vi "4_Analog_Meter_Reader(Inference)_(Input_From_File).vi"() -> ()   [LabVIEW 2020]
uses:
  Controls/Analog_Meter.ctl
  <vilib>/Ngene/Deep Learning Toolkit/Toolkit/NN_Network/Controls/NN_Save_Before_Destroy_Options.ctl
  <vilib>/Ngene/Deep Learning Toolkit/Toolkit/NN_Network/Controls/NN_Device.ctl
  <vilib>/Ngene/Deep Learning Toolkit/Toolkit/NN_Network/API/NN_Set_Input/3D/NN_Set_Input(3D_SGL_idx).vi
  <vilib>/Ngene/Deep Learning Toolkit/Toolkit/Deep_Learning_Toolkit_by_Ngene.lvlib
  <vilib>/ptbypt/NI_PtbyPt.lvlib
  <vilib>/vision/NI_Vision_Development_Module.lvlib
panel:
  out "Image Path":path=path "D:/working/Analog_Meter/Test/Images/0016.png"
  in  "File Path":path=path "D:/working/Analog_Meter/Test/Images/0016.png"
  out "Input":T1(plugin-control)
  out "Value":sgl=11.692846 format="%#.2g"
  out "Inference Time (ms)":dbl=0.008072819999924832 format="%#_3p"
  out "Prediction":T2=11.692846298217773 scale=0.0..140.0
  out "Inference Speed (FPS)":dbl=123.87245101579265 format="%#_3p"
  in  "Stop":bool
  in  "Network Configuration File Path":path=path "D:/Ngene/GitHub/deepltk_examples/3_Image_Processing/31_Image_Regression/working/Analog_Meter/Analog_Meter_net_cfg_24_01_29__19_35_37.cfg"
  in  "Weight File Path":path=path "D:/Ngene/GitHub/deepltk_examples/3_Image_Processing/31_Image_Regression/working/Analog_Meter/Analog_Meter_weights_24_01_29__19_35_37.bin"
  # "Instructions:\n1. Provide model files (.cfg and .bin).\n2. Run the VI\n3. Specify (Drag and Drop) an image from Test dataset in \"Input\" file path."
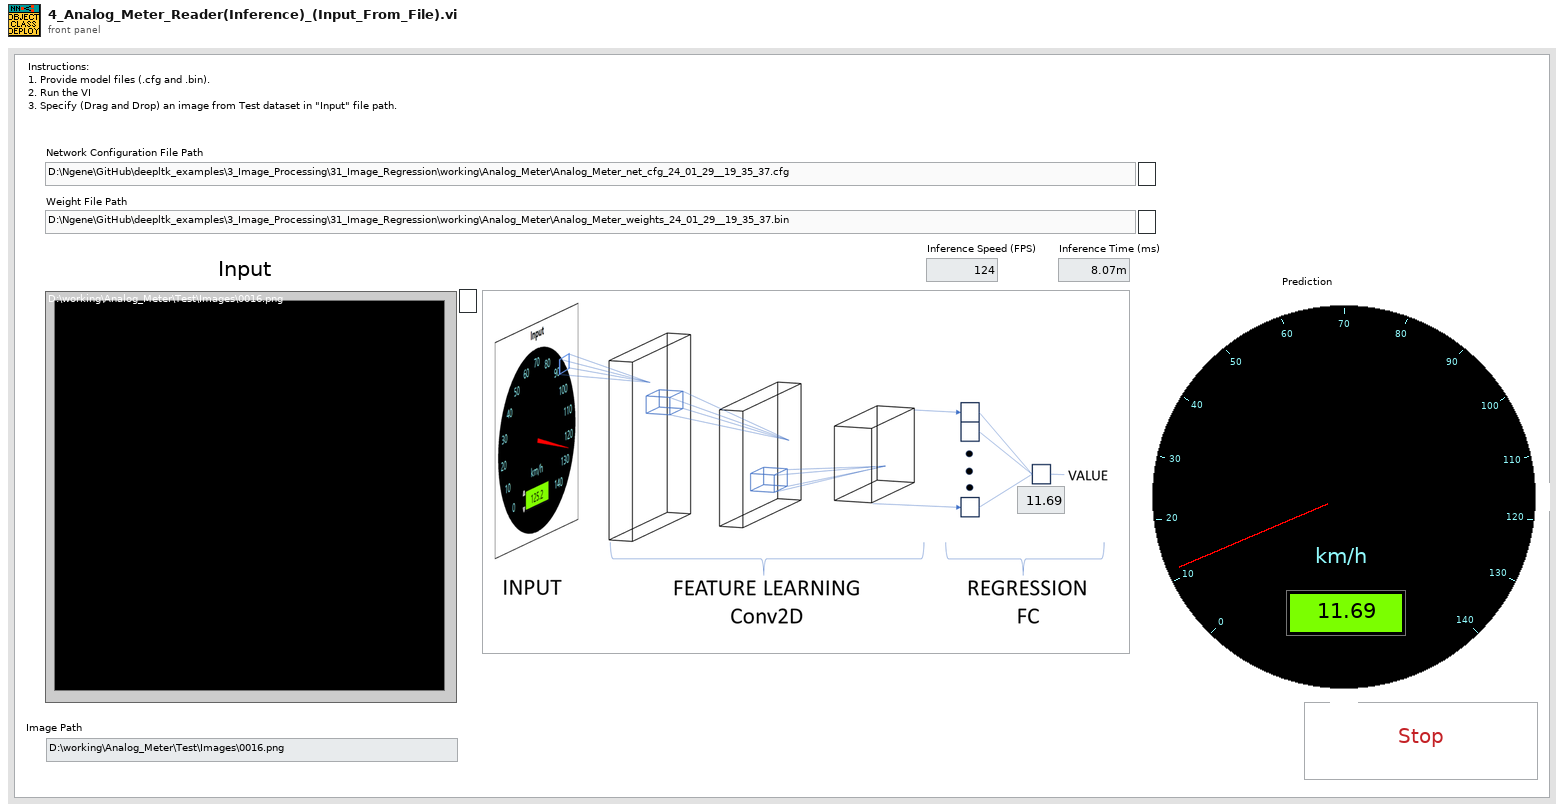
[diagram p1: front panel]
types:
  T1 = typedef "IMAQ Image.ctl" = refnum<image>
  T2 = typedef "Analog_Meter.ctl" = dbl
  T3 = typedef "Image Type" = u32
  T4 = typedef "Deep_Learning_Toolkit_by_Ngene.lvlib/NN_Device.ctl" = enum16{"CPU", "GPU"}
  T5 = typedef "Deep_Learning_Toolkit_by_Ngene.lvlib/NN_Save_Before_Destroy_Options.ctl" = cluster{"CFG?":bool, "Weights?":bool, "Render?":bool}
  T6 = typedef "Deep_Learning_Toolkit_by_Ngene.lvlib/NN_Config_Params.ctl" = cluster{"Name":string, "mBatch":i32, "NN_Train_Params":T7, "LR_Decay_Policy":T10, "Labels":string[], "Loss":T12}
  T7 = typedef "Deep_Learning_Toolkit_by_Ngene.lvlib/NN_Train_Params.ctl" = cluster{"Optimizer":T8, "Beta_1":sgl, "Beta_2":sgl, "Weight Decay(L1)":sgl, "Weight Decay(L2)":sgl, "Data_Sampling":T9}
  T8 = typedef "Deep_Learning_Toolkit_by_Ngene.lvlib/NN_Train_Optimizer.ctl" = enum16{"SGD", "Adam", "Adagrad", "Adadelta", "RMSProp", "Nesterov"}
  T9 = typedef "Deep_Learning_Toolkit_by_Ngene.lvlib/NN_Train_Data_Sampling.ctl" = enum16{"Random", "Sequential"}
  T10 = typedef "Deep_Learning_Toolkit_by_Ngene.lvlib/NN_LR_Policy_Cfg.ctl" = cluster{"Policy_Type":T11, "LR0":dbl, "k":sgl, "WarmUp_Policy":enum16{"Step", "Ramp"}, "WarmUp_Iter":i32, "WarmUp_Ratio":sgl}
  T11 = typedef "Deep_Learning_Toolkit_by_Ngene.lvlib/NN_LR_Policy_Type.ctl" = enum16{"Manual", "Step", "Exp", "1/t"}
  T12 = typedef "Deep_Learning_Toolkit_by_Ngene.lvlib/NN_Loss_Config_Params.ctl" = cluster{"Loss_Type":T13, "Loss_Conf_Params":variant}
  T13 = typedef "Deep_Learning_Toolkit_by_Ngene.lvlib/NN_Loss_Type.ctl" = enum16{"None", "MSE", "CrossEntropy", "YOLO_v2", "YOLO_v4"}
  T14 = typedef "Deep_Learning_Toolkit_by_Ngene.lvlib/NN_Layer_Config_Params.ctl" = cluster{"Layer_Type":T15, "Layer_Conf_Params":variant, "Input Layers":string[]}
  T15 = typedef "Deep_Learning_Toolkit_by_Ngene.lvlib/NN_Layer_Type.ctl" = enum16{"Input1D", "Input3D", "Conv1D", "Conv2D", "Conv2D_Adv", "MaxPool", "AvgPool", "UpSample", "DropOut3D", "ShortCut", "Concat", "SoftMax3D", "FC", "DropOut", "Softmax", "Flatten", "YOLO_v2", "YOLO_v4", "Activation", "BatchNormalization", "Unsupported"}
  T16 = typedef "Deep_Learning_Toolkit_by_Ngene.lvlib/NN.ctl" = cluster{"Name":string, "No of Layers":i32, "mBatch":i32, "Layers":T17[], "Dimty":T18, "Dims_In":T19, "Dims_Out":T19, "Working_Dir":path, "Train?":bool, "Train_Params":T7, "LR_Update_Policy":T10, "Session Data":T20, "Ground_truth":T21, "NNg_hdls":T22, "NN_Device":T4, "GPU Id":i32, "Labels":string[], "Receptive Field":T23[], "Loss_Type":T13, "Loss_Cfg_Prms":variant, "NNG_WS":T24}
  T17 = typedef "Deep_Learning_Toolkit_by_Ngene.lvlib/NN_Layer_ref.ctl" = refnum<data-value>
  T18 = typedef "Deep_Learning_Toolkit_by_Ngene.lvlib/NN_In_Out_Dim-ty.ctl" = enum8{"In1D_Out1D", "In3D_Out1D", "In3D_Out3D", "In3D_OutBBox"}
  T19 = typedef "Deep_Learning_Toolkit_by_Ngene.lvlib/NN_Dims(C,H,W).ctl" = cluster{"C":i32, "H":i32, "W":i32}
  T20 = typedef "Deep_Learning_Toolkit_by_Ngene.lvlib/NN_Train_Session_Data.ctl" = cluster{"Epochs":sgl, "Tot_Iter":i32, "LR":sgl, "LR_iter":i32}
  T21 = typedef "Deep_Learning_Toolkit_by_Ngene.lvlib/NN_Ground_truth.ctl" = cluster{"Y":variant}
  T22 = typedef "Deep_Learning_Toolkit_by_Ngene.lvlib/nng_cuda_handles.ctl" = cluster{"cudnn":u64, "cublas":u64, "stream":u64, "curand":u64}
  T23 = typedef "Deep_Learning_Toolkit_by_Ngene.lvlib/NN_Dims(V,H).ctl" = cluster{"V":i32, "H":i32}
  T24 = typedef "Deep_Learning_Toolkit_by_Ngene.lvlib/NNG_WS.ctl" = cluster{"NNG_WS_Mem":T25, "Max_WS_Size":i64}
  T25 = typedef "Deep_Learning_Toolkit_by_Ngene.lvlib/NNg_WS_Mem_DVR.ctl" = refnum<data-value>
  T26 = typedef "Deep_Learning_Toolkit_by_Ngene.lvlib/NN_Layer.ctl" = cluster{"Name":string, "Layer_Data":variant, "Layer_Type":T15, "Dims_In":T19, "Layers_In":variant, "Dims_Out":T19, "Layers_Out":variant, "Metrics":T27, "GPU_Data":variant, "mBatch":i32, "NN_Device":T4, "NNg_hdls":T22, "Train?":bool, "Dimty":T28, "RecptField":T29}
  T27 = typedef "Deep_Learning_Toolkit_by_Ngene.lvlib/NN_Layer_Metrics.ctl" = cluster{"Data":dbl, "Params":dbl, "Ops":dbl}
  T28 = typedef "Deep_Learning_Toolkit_by_Ngene.lvlib/NN_Layer_Dimty.ctl" = enum16{"1D", "3D"}
  T29 = typedef "Deep_Learning_Toolkit_by_Ngene.lvlib/NN_Layer_RF_State.ctl" = cluster{"Dims":T23, "J":T23}
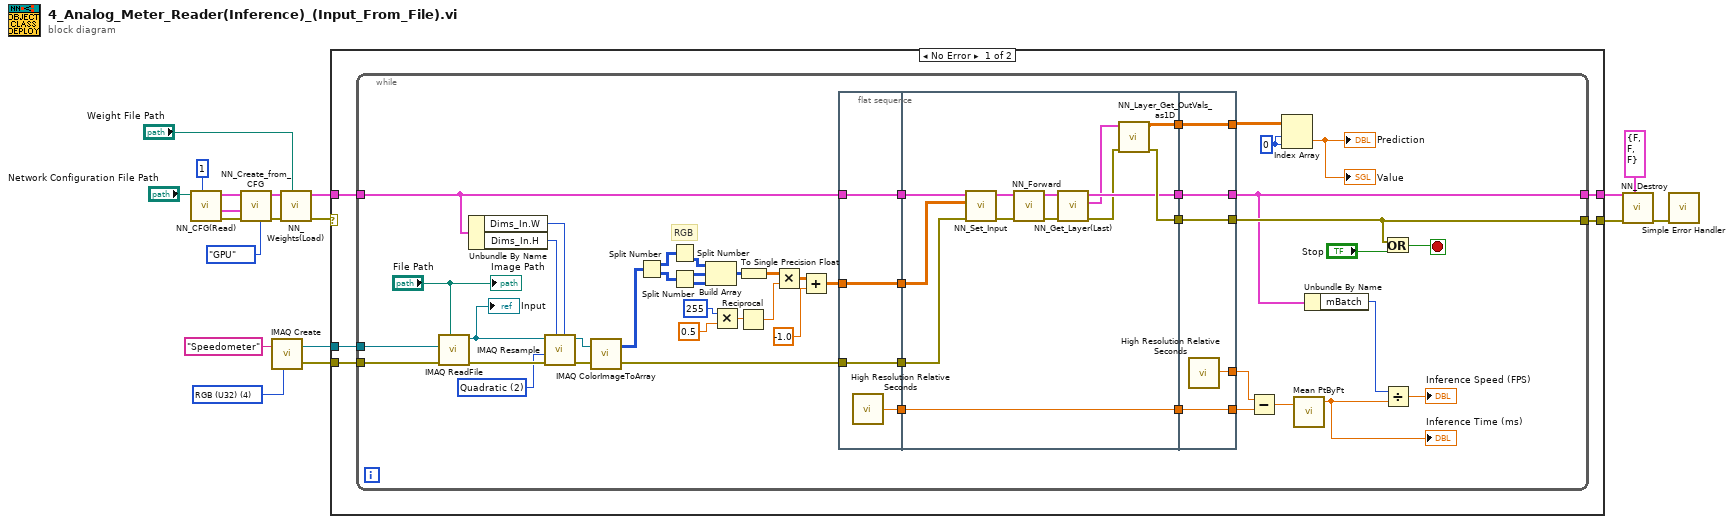
[diagram p0: block diagram]
diagram:
  w2 = T3 4 items=["Grayscale (U8)", "Grayscale (I16)", "Grayscale (SGL)", "Complex (CSG)", "RGB (U32)", "HSL (U32)", "RGB (U64)", "Grayscale (U16)"] ("Image Type")
  n1 = call <vilib>:"NN_CFG(Read).vi"("mBatch"=1, "CFG file path"="Network Configuration File Path") -> ("error out"=w19:errorcluster, "Net_Cfg"=w8:T6, "Layer_Cfg"=w12:T14[])  [unwired: 7 in]
  n2 = call <vilib>:"NN_Create_from_CFG.vi"("NN_Device"=NN_Device."GPU", "error in (no error)"=w19, "Net_Cfg"=w8, "Layer_Cfg"=w12) -> ("error out"=w14:errorcluster, "NN out"=w11:T16)  [unwired: 6 in]
  n3 = call "IMAQ Create"("Image Name"="Speedometer", "Image Type"=w2) -> ("New Image"=w4:T1, "error out"=w3:errorcluster)  [unwired: 3 in]
  n4 = call <vilib>:"NN_Weights(Load).vi"("Weight File Path"="Weight File Path", "error in (no error)"=w14, "NN in"=w11) -> ("error out"=w9:errorcluster, "NN out"=w10:T16)  [unwired: 7 in]
  n5 = case shown="No Error" w9 {
    selector: w9 -> [_ w95]
    tunnel: w10 -> [w24 w96]
    tunnel: [w23 w96] -> w17
    tunnel: [w22 w95] -> w16
    tunnel: w4 -> [w21 _]
    tunnel: w3 -> [w20 _]
    frame No Error {
      n6 = while {
        tunnel: w24 -> [w33]
        tunnel: [w69] -> w23
        tunnel: [w70] -> w22
        tunnel: w21 -> [w36]
        tunnel: w20 -> [w35]
        stop <- w71 stop-if-true
        w26 = u32 2 items=["Zero Order", "Bi-Linear", "Quadratic", "Cubic Spline"] ("Interpolation Type")
        w59 = 0 ("disabled index (col)")
        # "RGB"
        n7 = call "IMAQ ReadFile"("File Path"="File Path", "error in (no error)"=w35, "Image"=w36) -> ("error out"=w31:errorcluster, "Image Out"=w28:T1)  [unwired: 4 in, 3 out]
        "Input" <- w28
        n8 = Unbundle By Name(w33) -> ("Dims_In.W"=w30:i32, "Dims_In.H"=w29:i32)
        n9 = call "IMAQ Resample"("X Resolution"=w30, "Y Resolution"=w29, "error in (no error)"=w31, "Interpolation Type"=w26, "Image Src"=w28) -> ("error out"=w32:errorcluster, "Image Dst Out"=w27:T1)  [unwired: 5 in]
        n10 = call "IMAQ ColorImageToArray"("Image"=w27, "error in (no error)"=w32) -> ("Image Pixels (U32)"=w37:u32[][], "error out"=w34:errorcluster)  [unwired: 2 in, 1 out]
        n11 = Split Number(x=w37) -> (hi(x)=w57:u16[][], lo(x)=w58:u16[][])
        n12 = Split Number(x=w57) -> (lo(x)=w55:u8[][])  [unwired: 1 out]
        n13 = Split Number(x=w58) -> (hi(x)=w54:u8[][], lo(x)=w53:u8[][])
        n14 = Build Array(w55, w54, w53) -> (w56:u8[][][])
        n15 = Multiply(x=u16 255 ("dimension size"), y=sgl 0.5 ("dimension size")) -> (x*y=w51:sgl)
        n16 = Reciprocal(x=w51) -> (1/x=w52:sgl)
        n17 = To Single Precision Float(number=w56) -> (single precision float=w46:sgl[][][])
        n18 = Multiply(x=w46, y=w52) -> (x*y=w50:sgl[][][])
        n19 = Add(x=w50, y=sgl -1.0 ("dimension size")) -> (x+y=w44:sgl[][][])
        n20 = flat-sequence {
          tunnel: w34 -> [w75]
          tunnel: w33 -> [w76]
          tunnel: [w76] -> w67
          tunnel: [w75] -> w66
          tunnel: [w74] -> w45
          tunnel: w44 -> [w74]
          tunnel: [w73] -> w41
          tunnel: w67 -> [w88]
          tunnel: w66 -> [w79]
          tunnel: [w89] -> w65
          tunnel: [w87] -> w64
          tunnel: [w86] -> w63
          tunnel: w45 -> [w78]
          tunnel: [w77] -> w42
          tunnel: w41 -> [w77]
          tunnel: [w92] -> w69
          tunnel: [w93] -> w70
          tunnel: [w94] -> w72
          tunnel: w65 -> [w94]
          tunnel: w64 -> [w93]
          tunnel: w63 -> [w92]
          tunnel: [w91] -> w62
          tunnel: [w90] -> w43
          tunnel: w42 -> [w90]
          frame #0 {
            n21 = call <vilib>:"High Resolution Relative Seconds.vi"() -> ("relative seconds"=w73:dbl)
          }
          frame #1 {
            n22 = call-poly <vilib>:"NN_Set_Input.vi"("error in (no error)"=w79, "Data_In(3D_SGL)"=w78, "NN in"=w88) -> ("error out"=w83:errorcluster, "NN out"=w82:T16)  [unwired: 7 in]
            n23 = call <vilib>:"NN_Forward.vi"("error in (no error)"=w83, "NN in"=w82) -> ("error out"=w81:errorcluster, "NN out"=w80:T16)  [unwired: 6 in, 2 out]
            n24 = call <vilib>:"NN_Get_Layer(Last).vi"("error in (no error)"=w81, "NN in"=w80) -> ("error out"=w85:errorcluster, "Last_Layer"=w84:T26, "NN out"=w86:T16)  [unwired: 6 in, 1 out]
            n25 = call <vilib>:"NN_Layer_Get_OutVals_as1D.vi"("error in (no error)"=w85, "Layer"=w84) -> ("error out"=w87:errorcluster, "Out(as1D)"=w89:sgl[][])  [unwired: 8 in]
          }
          frame #2 {
            n26 = call <vilib>:"High Resolution Relative Seconds.vi"() -> ("relative seconds"=w91:dbl)
          }
        }
        n27 = Subtract(x=w62, y=w43) -> (x-y=w39:dbl)
        n28 = Index Array(array=w72, index (row)=w59, index (col)=w59) -> (element=→"Prediction" →"Value":sgl)
        n29 = call <vilib>:"Mean PtByPt.vi"("x"=w39) -> ("mean"=w38:dbl)  [unwired: 3 in, 1 out]
        "Inference Time (ms)" <- w38
        n30 = Unbundle By Name(w69) -> ("mBatch"=w68:i32)
        n31 = Or(x=w70, y="Stop") -> (x .or. y?=w71:bool)
        n32 = Divide(x=w68, y=w38) -> (x/y=→"Inference Speed (FPS)":dbl)
        "Image Path" <- "File Path"
      }
    }
    frame Error {
    }
  }
  n33 = call <vilib>:"NN_Destroy.vi"("Save (T, T, T)"=T5 {"CFG?"=FALSE, "Weights?"=FALSE, "Render?"=FALSE} ("Save_Config"), "error in (no error)"=w16, "NN in"=w17) -> ("error out"=w1:errorcluster)  [unwired: 7 in, 1 out]
  n34 = call <vilib>:"Simple Error Handler.vi"("error in (no error)"=w1) -> ()  [unwired: 4 in, 5 out]
